vi "Close Client.vi"(8 "Error In":errorcluster, 11 "Client Ref":refnum<k24>) -> (0 "Error Out":errorcluster)   [LabVIEW 2014, in "SSL Lib.lvlib"]
doc: "VI Function: This VI closes the client reference.\n\nVI Version: 1.0\n\nVI Author: Runjhun Agarwal"
uses:
  <userlib>/SSL Library/SSL Lib.lvlib
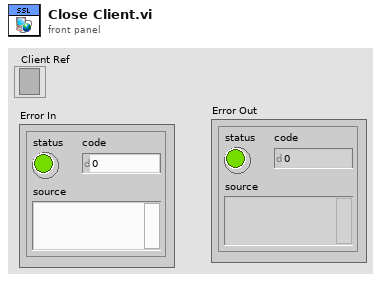
[diagram p1: front panel]
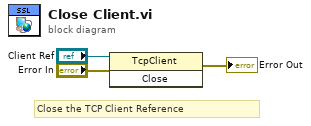
[diagram p0: block diagram]
diagram:
  # "Close the TCP Client Reference"
  n1 = invoke class="TcpClient" method="Close"(reference="Client Ref", error in="Error In") -> (error out=→"Error Out":errorcluster)  [unwired: 1 in, 2 out]
